vi "Reserve SCOPE Session.vi"(8 "error in (no error)":errorcluster, 9 "Measurement Configuration In":T1={"Start Freq."=100.0, "Freq. Step"=10.0, "Stop Frequ."=1000000.0, "Amplitude"=1.0, "Timing (ms)"=0, "Vin_signal"="Vin_signal", "Vin_measure"="Vin_measure", "Vout_measure"="Vout_measure"} {"Stop Frequ." format="%#_6p"; "Freq. Step" format="%#_6p"; "Start Freq." format="%#_6p"}, 11 "Measurement Context":refnum<class "MeasurementContext.lvclass">) -> (0 "error out":errorcluster, 1 "Measurement Configuration Out":T1={"Start Freq."=100.0, "Freq. Step"=10.0, "Stop Frequ."=1000000.0, "Amplitude"=1.0, "Timing (ms)"=0, "Vin_signal"="Vin_signal", "Vin_measure"="Vin_measure", "Vout_measure"="Vout_measure"} {"Stop Frequ." format="%#_6p"; "Freq. Step" format="%#_6p"; "Start Freq." format="%#_6p"}, 2 "Session":T2, 3 "Measurement Context out":refnum<class "MeasurementContext.lvclass">, 5 "scope_out":refnum<k15>)   [LabVIEW 2023, in "LabVIEW Bodeplot Summit.lvlib"]
doc: "Reserve Runtime Session for Fgen"
uses:
  LabVIEW Bodeplot Summit.lvlib
  <vilib>/MeasurementLink/MeasurementLink Measurement Server/Classes/MeasurementContext/MeasurementContext.lvclass
  Measurement Configuration.ctl
  Session Info.ctl
  <vilib>/gRPC/LabVIEW gRPC Library/Shared/grpcId.ctl
  <vilib>/MeasurementLink/MeasurementLink Session Management Client/RPC Messages/ni_measurementlink_sessionmanagement_v1_ReserveSessionsResponse.ctl
  <vilib>/MeasurementLink/MeasurementLink Session Management Client/RPC Messages/ni_measurementlink_sessionmanagement_v1_SessionInformation.ctl
  <vilib>/MeasurementLink/MeasurementLink Session Management Client/RPC Messages/nidevice_grpc_Session.ctl
  <vilib>/MeasurementLink/MeasurementLink Session Management Client/RPC Messages/ni_measurementlink_sessionmanagement_v1_ChannelMapping.ctl
  <vilib>/MeasurementLink/MeasurementLink Session Management Client/RPC Messages/ni_measurementlink_sessionmanagement_v1_ReserveSessionsRequest.ctl
  <vilib>/MeasurementLink/MeasurementLink Session Management Client/RPC Messages/ni_measurementlink_PinMapContext.ctl
  <vilib>/MeasurementLink/MeasurementLink Discovery Client/RPC Messages/ni_measurementlink_discovery_v1_ServiceLocation.ctl
  <vilib>/MeasurementLink/MeasurementLink Discovery Client/RPC Messages/ni_measurementlink_discovery_v1_ResolveServiceRequest.ctl
  <instrlib>/niScope/niScope gRPC Device Server.ctl
  <vilib>/MeasurementLink/MeasurementLink Measurement Server/MeasurementLink Measurement Server.lvlib
  <vilib>/MeasurementLink/MeasurementLink Session Management Client/MeasurementLink Session Management Client.lvlib
  <vilib>/MeasurementLink/MeasurementLink Discovery Client/MeasurementLink Discovery Client.lvlib
  <vilib>/gRPC/LabVIEW gRPC Library/grpc-lvsupport-release.lvlib
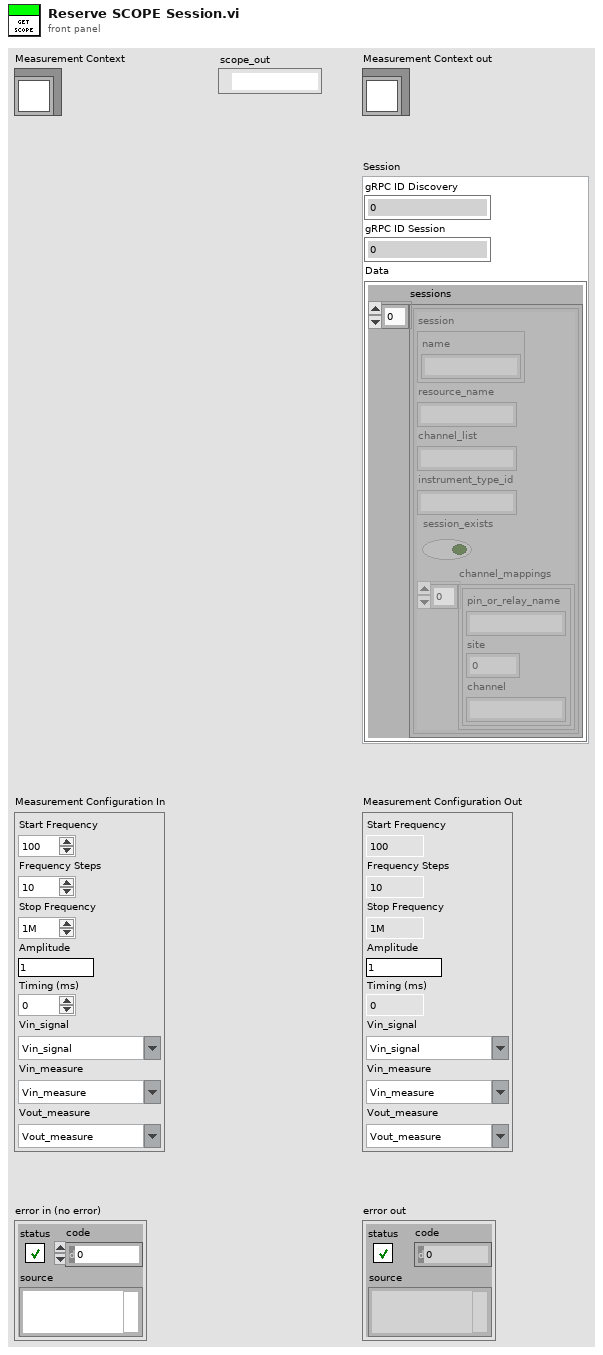
[diagram p1: front panel]
types:
  T1 = typedef "LabVIEW Bodeplot Summit.lvlib/Measurement Configuration.ctl" = cluster{"Start Freq.":dbl, "Freq. Step":dbl, "Stop Frequ.":dbl, "Amplitude":dbl, "Timing (ms)":u32, "Vin_signal":string, "Vin_measure":string, "Vout_measure":string}
  T2 = typedef "LabVIEW Bodeplot Summit.lvlib/Session Info.ctl" = cluster{"gRPC ID Discovery":T3, "gRPC ID Session":T3, "Data":T4}
  T3 = typedef "grpc-lvsupport-release.lvlib/grpcId.ctl" = u64
  T4 = typedef "MeasurementLink Session Management Client.lvlib/ni_measurementlink_sessionmanagement_v1_ReserveSessionsResponse.ctl" = cluster{"sessions":T5[]}
  T5 = typedef "MeasurementLink Session Management Client.lvlib/ni_measurementlink_sessionmanagement_v1_SessionInformation.ctl" = cluster{"session":T6, "resource_name":string, "channel_list":string, "instrument_type_id":string, "session_exists":bool, "channel_mappings":T7[]}
  T6 = typedef "MeasurementLink Session Management Client.lvlib/nidevice_grpc_Session.ctl" = cluster{"name":string}
  T7 = typedef "MeasurementLink Session Management Client.lvlib/ni_measurementlink_sessionmanagement_v1_ChannelMapping.ctl" = cluster{"pin_or_relay_name":string, "site":i32, "channel":string}
  T8 = typedef "MeasurementLink Discovery Client.lvlib/ni_measurementlink_discovery_v1_ServiceLocation.ctl" = cluster{"location":string, "insecure_port":string, "ssl_authenticated_port":string}
  T9 = typedef "MeasurementLink Session Management Client.lvlib/ni_measurementlink_sessionmanagement_v1_ReserveSessionsRequest.ctl" = cluster{"pin_map_context":T10, "pin_or_relay_names":string[], "instrument_type_id":string, "timeout_in_milliseconds":i32}
  T10 = typedef "MeasurementLink Session Management Client.lvlib/ni_measurementlink_PinMapContext.ctl" = cluster{"pin_map_id":string, "sites":i32[]}
  T11 = typedef "MeasurementLink Measurement Server.lvlib/PinMapContext.ctl" = cluster{"pin_map_id":string, "sites":i32[]}
  T12 = typedef "MeasurementLink Discovery Client.lvlib/ni_measurementlink_discovery_v1_ResolveServiceRequest.ctl" = cluster{"provided_interface":string, "service_class":string}
  T13 = typedef "niScope gRPC Device Server.ctl" = cluster{"session name":string, "address (localhost)":string, "port (31763)":u32}
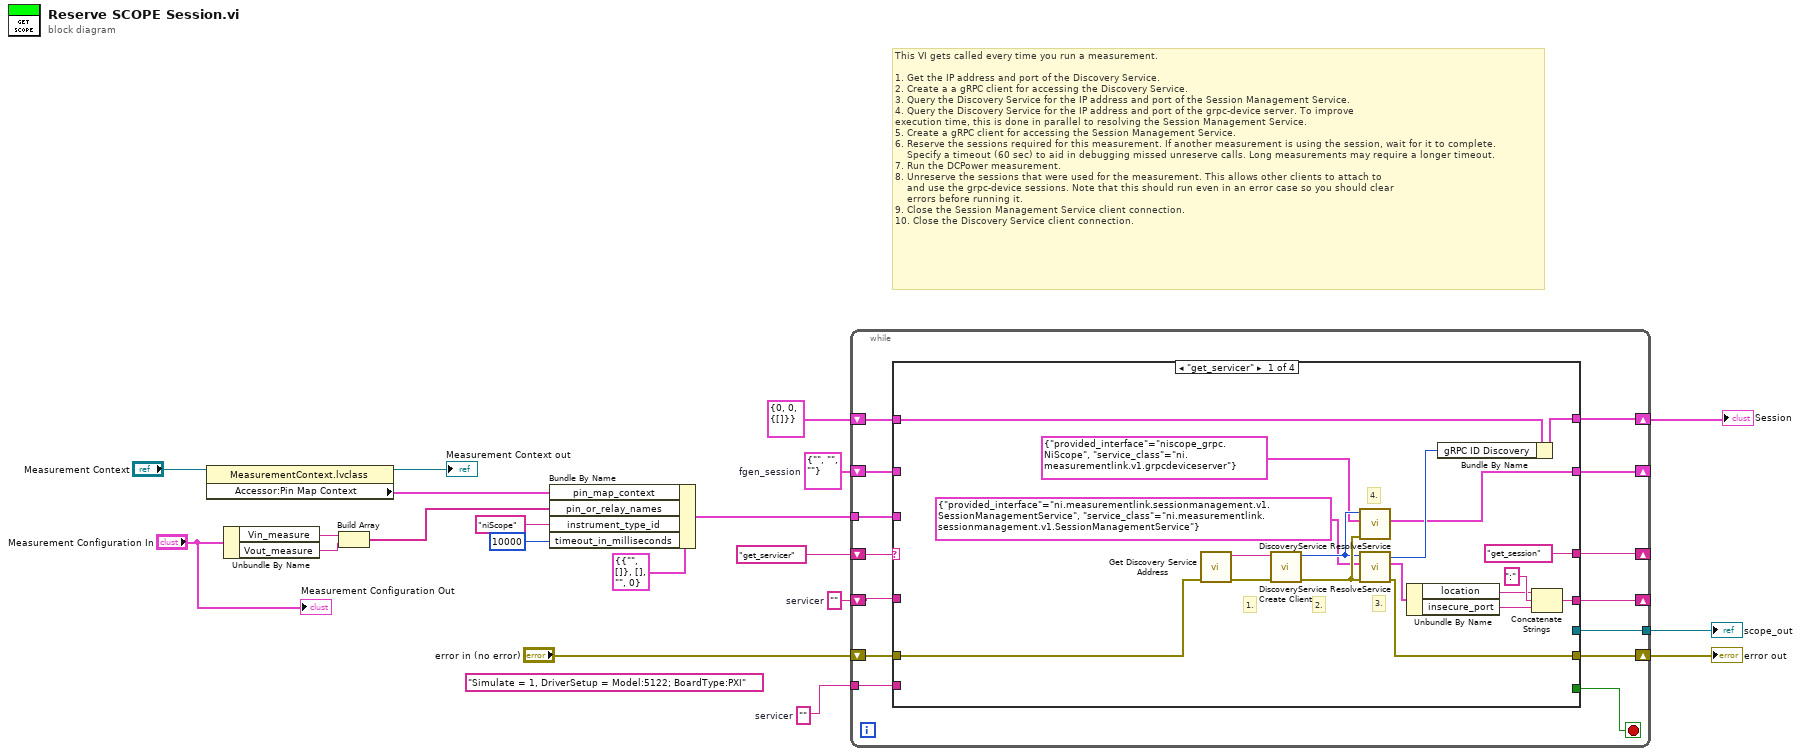
[diagram p0: block diagram]
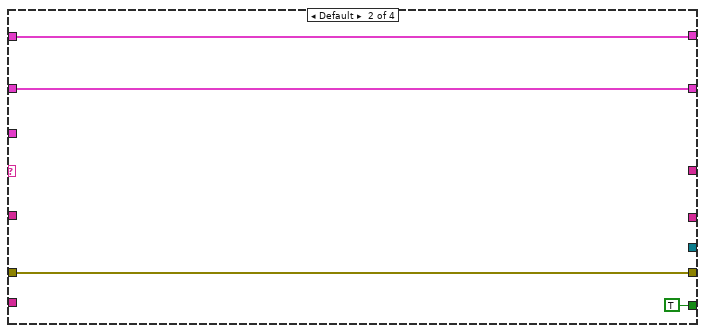
[diagram p2: hidden frame]
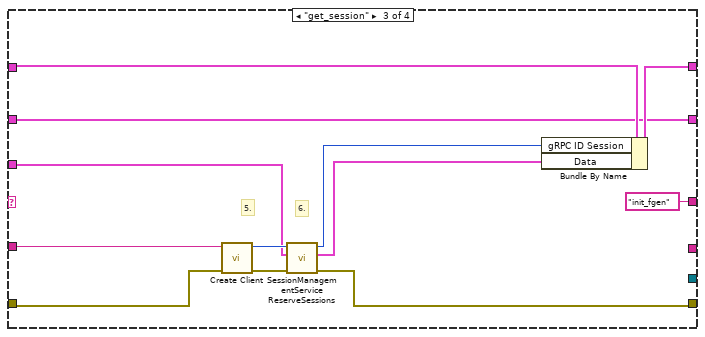
[diagram p3: hidden frame]
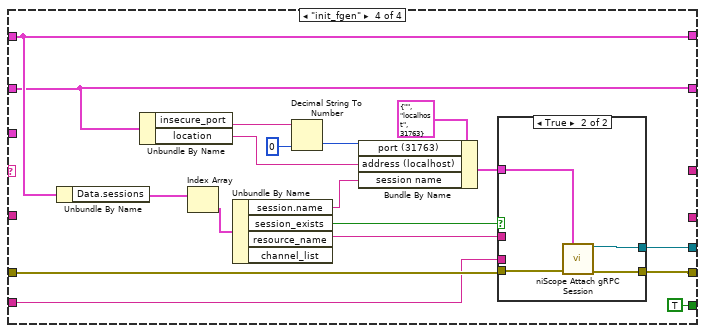
[diagram p4: hidden frame]
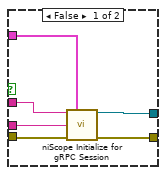
[diagram p5: hidden frame]
diagram:
  w1 = ""  # servicer
  (unwired) "Simulate = 1, DriverSetup = Model:5122; BoardType:PXI"
  w6 = T8 {"location"="", "insecure_port"="", "ssl_authenticated_port"=""}  # fgen_session
  w9 = ""  # servicer
  # "This VI gets called every time you run a measurement.\n\n1. Get the IP address and port of the Discovery Service.\n2. Create a a gRPC client for accessing the Discovery Service.\n3. Query the Discovery Service for the IP address and port of the Session Management Service.\n4. Query the Discovery Service for the IP address and port of the grpc-device server. To improve \nexecution time, this is done in parallel to resolving the Session Management Service.\n5. Create a gRPC client for accessing the Session Management Service.\n6. Reserve the sessions required for this measurement. If another measurement is using the session, wait for it to complete. \n    Specify a timeout (60 sec) to aid in debugging missed unreserve calls. Long measurements may require a longer timeout.\n7. Run the DCPower measurement.\n8. Unreserve the sessions that were used for the measurement. This allows other clients to attach to\n    and use the grpc-device sessions. Note that this should run even in an error case so you should clear \n    errors before running it.\n9. Close the Session Management Service client connection.\n10. Close the Discovery Service client connection."
  n1 = property class="MeasurementContext.lvclass"(reference="Measurement Context") -> (reference out=→"Measurement Context out":refnum<class "MeasurementContext.lvclass">, "Accessor:Pin Map Context"=w18:T11)  [unwired: 1 in, 1 out]
  n2 = Unbundle By Name("Measurement Configuration In") -> ("Vin_measure"=w14:string, "Vout_measure"=w3:string)
  n3 = Build Array(w14, w3) -> (w13:string[])
  n4 = Bundle By Name(cluster=T9 {"pin_map_context"={"pin_map_id"="", "sites"=[]}, "pin_or_relay_names"=[], "instrument_type_id"="", "timeout_in_milliseconds"=0} ("Request Data"), "pin_map_context"=w18, "pin_or_relay_names"=w13, "instrument_type_id"="niScope" ("Instrument Type Id"), "timeout_in_milliseconds"=10000) -> (w8:T9)
  n5 = while {
    shift-right: [w28] -> _
    shift-left: "get_servicer" -> [w34]
    shift-right: [w30] -> w7
    shift-left: T2 {"gRPC ID Discovery"=0, "gRPC ID Session"=0, "Data"={"sessions"=[]}} ("Session") -> [w31]
    shift-right: [w29] -> _
    shift-left: w9 -> [w27]
    shift-right: [w32] -> w4
    shift-left: "error in (no error)" -> [w33]
    tunnel: w8 -> [w26]
    shift-right: [w25] -> _
    shift-left: w6 -> [w24]
    tunnel: w1 -> [w23]
    tunnel: [w22] -> w5
    stop <- w21 stop-if-true
    n6 = case shown="\"get_servicer\"" w34 {
      tunnel: w33 -> [w46 w54 w65 w74]
      tunnel: [w45 w54 w60 w73] -> w32
      tunnel: w31 -> [w44 w56 w63 w85]
      tunnel: [w43 w56 w61 w85] -> w30
      tunnel: [w37 _ _ _] -> w29
      tunnel: ["get_session" _ "init_fgen" _] -> w28
      tunnel: w27 -> [_ _ w66 _]
      tunnel: w26 -> [_ _ w64 _]
      tunnel: [w35 w55 w57 w75] -> w25
      tunnel: w24 -> [_ w55 w57 w75]
      tunnel: w23 -> [_ _ _ w72]
      tunnel: [_ _ _ w71] -> w22
      tunnel: [_ TRUE _ TRUE] -> w21
      frame "get_servicer" {
        # "4."
        # "3."
        # "2."
        # "1."
        n7 = call <vilib>:"Get Discovery Service Address.vi"("error in"=w46) -> ("error out"=w49:errorcluster, "address"=w50:string)  [unwired: 9 in]
        n8 = call <vilib>:"Create Client.vi"("error in"=w49, "address"=w50) -> ("error out"=w52:errorcluster, "gRPC ID Out"=w51:T3)  [unwired: 8 in]
        n9 = call <vilib>:"DiscoveryService ResolveService.vi"("error in"=w52, "Request Data"=T12 {"provided_interface"="niscope_grpc.NiScope", "service_class"="ni.measurementlink.v1.grpcdeviceserver"}, "gRPC ID"=w51) -> ("Response Data"=w35:T8)  [unwired: 6 in, 2 out]
        n10 = call <vilib>:"DiscoveryService ResolveService.vi"("error in"=w52, "Request Data"=T12 {"provided_interface"="ni.measurementlink.sessionmanagement.v1.SessionManagementService", "service_class"="ni.measurementlink.sessionmanagement.v1.SessionManagementService"}, "gRPC ID"=w51) -> ("error out"=w45:errorcluster, "Response Data"=w40:T8, "gRPC ID out"=w42:T3)  [unwired: 6 in]
        n11 = Unbundle By Name(w40) -> ("location"=w39:string, "insecure_port"=w38:string)
        n12 = Bundle By Name(cluster=w44, "gRPC ID Discovery"=w42) -> (w43:T2)
        n13 = Concatenate Strings(w39, ":" ("string"), w38) -> (w37:string)
      }
      frame Default {
      }
      frame "get_session" {
        # "6."
        # "5."
        n14 = call <vilib>:"Create Client.vi"("error in"=w65, "address"=w66) -> ("error out"=w68:errorcluster, "gRPC ID Out"=w67:T3)  [unwired: 8 in]
        n15 = call <vilib>:"SessionManagementService ReserveSessions.vi"("error in"=w68, "Request Data"=w64, "gRPC ID"=w67) -> ("error out"=w60:errorcluster, "Response Data"=w62:T4, "gRPC ID out"=w59:T3)  [unwired: 6 in]
        n16 = Bundle By Name(cluster=w63, "gRPC ID Session"=w59, "Data"=w62) -> (w61:T2)
      }
      frame "init_fgen" {
        n17 = Unbundle By Name(w85) -> ("Data.sessions"=w86:T5[])
        n18 = Unbundle By Name(w75) -> ("insecure_port"=w82:string, "location"=w81:string)
        n19 = Index Array(array=w86) -> (element=w76:T5)  [unwired: 1 in]
        n20 = Unbundle By Name(w76) -> ("session.name"=w80:string, "session_exists"=w78:bool, "resource_name"=w84:string)  [unwired: 1 out]
        n21 = Decimal String To Number(string=w82, default (0L)=u32 0 ("Port (31763)")) -> (number=w83:u32)  [unwired: 1 in, 1 out]
        n22 = Bundle By Name(cluster=T13 {"session name"="", "address (localhost)"="localhost", "port (31763)"=31763} ("gRPC options"), "port (31763)"=w83, "address (localhost)"=w81, "session name"=w80) -> (w79:T13)
        n23 = case shown="True" w78 {
          tunnel: w74 -> [w88 w96]
          tunnel: w79 -> [w91 w95]
          tunnel: [w90 w94] -> w73
          tunnel: [w92 w93] -> w71
          tunnel: w84 -> [w89 _]
          tunnel: w72 -> [w87 _]
          frame False {
            n24 = call <instrlib>:"niScope Initialize for gRPC Session.vi"("resource name"=w89, "gRPC options"=w91, "option string"=w87, "error in"=w88) -> ("instrument handle"=w92:refnum<k15>, "error out"=w90:errorcluster)  [unwired: 10 in]
          }
          frame True {
            n25 = call <instrlib>:"niScope Attach gRPC Session.vi"("gRPC options"=w95, "error in"=w96) -> ("instrument handle"=w93:refnum<k15>, "error out"=w94:errorcluster)  [unwired: 12 in]
          }
        }
      }
    }
  }
  "error out" <- w4
  "scope_out" <- w5
  "Session" <- w7
  "Measurement Configuration Out" <- "Measurement Configuration In"
